vi "CLSUIP_GetOverlayImageData.vi"(2 "error in (no error)":errorcluster, 3 "Access":T1) -> (0 "error out":errorcluster, 1 "image data":T2)   [LabVIEW 2021, in "MemberVICreation.lvlib"]
uses:
  <resource>/Framework/Providers/LVClassLibrary/NewAccessors/MemberVICreation.lvlib
  <vilib>/picture/picture.llb/imagedata.ctl
  <resource>/Framework/Providers/LVClassLibrary/NewAccessors/CLSUIP_Access.ctl
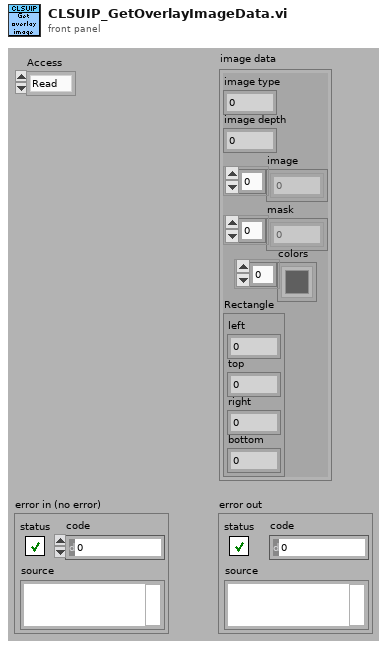
[diagram p1: front panel]
types:
  T1 = typedef "MemberVICreation.lvlib/CLSUIP_Access.ctl" = enum16{"Read", "Write", "R/W"}
  T2 = typedef "imagedata.ctl" = cluster{"image type":i32, "image depth":i32, "image":u8[], "mask":u8[], "colors":u32[], "Rectangle":cluster{"left":i16, "top":i16, "right":i16, "bottom":i16}}
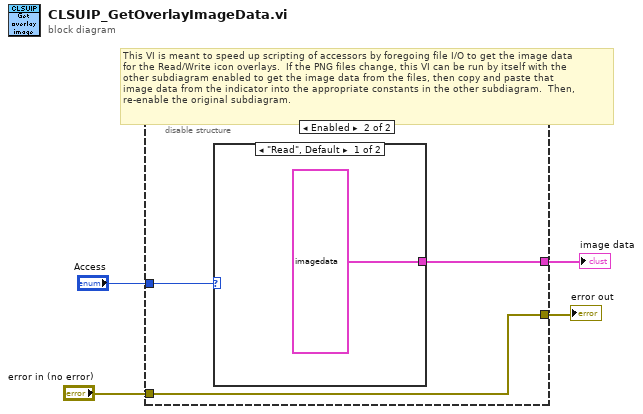
[diagram p0: block diagram]
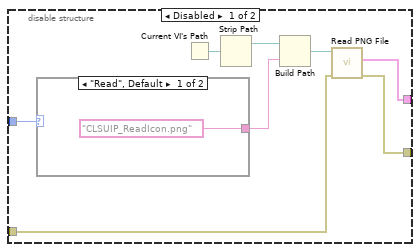
[diagram p2: hidden frame]
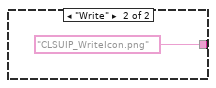
[diagram p3: hidden frame]
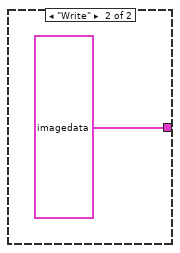
[diagram p4: hidden frame]
diagram:
  # "This VI is meant to speed up scripting of accessors by foregoing file I/O to get the image data\nfor the Read/Write icon overlays.  If the PNG files change, this VI can be run by itself with the\nother subdiagram enabled to get the image data from the files, then copy and paste that\nimage data from the indicator into the appropriate constants in the other subdiagram.  Then,\nre-enable the original subdiagram."
  n1 = disable-structure shown="Enabled" {
    disable-tunnel: [w12 w15] -> w4
    disable-tunnel: [w11 w16] -> w3
    disable-tunnel: "error in (no error)" -> [w9 w15]
    disable-tunnel: "Access" -> [w7 w17]
    frame Disabled {
      n2 = case shown="\"Read\", Default" w7 {
        tunnel: ["CLSUIP_ReadIcon.png" "CLSUIP_WriteIcon.png"] -> w8
        frame "Read", Default {
        }
        frame "Write" {
        }
      }
      n3 = Current VI's Path() -> (path=w5:path)
      n4 = Strip Path(path=w5) -> (stripped path=w6:path)  [unwired: 1 out]
      n5 = Build Path(base path=w6, name or relative path=w8) -> (appended path=w10:path)
      n6 = call <vilib>:"Read PNG File.vi"("error in (no error)"=w9, "path to PNG file"=w10) -> ("error out"=w12:errorcluster, "image data"=w11:T2)  [unwired: 7 in, 1 out]
    }
    frame Enabled {
      n7 = case shown="\"Read\", Default" w17 {
        tunnel: [T2 {"image type"=0, "image depth"=24, "image"=[255, 255, 255, 255, 255, 255, 255, 255, 255, 255, 255, 255, 255, 255, 255, 0, 0, 0, 0, 0, 0, 255, 255, 255, 255, 255, 255, 255, 255, 255, 255, 255, 255, 255, 255, 255, 255, 255, 255, 0, 0, 0, 0, 0, 0, 255, 255, 255, 255, 255, 255, 255, 255, 255, 255, 255, 255, 255, 255, 255, 0, 0, 0, 255, 255, 255, 255, 255, 255, 0, 0, 0, 255, 255, 255, 255, 255, 255, 255, 255, 255, 255, 255, 255, 0, 0, 0, 255, 255, 255, 255, 255, 255, 0, 0, 0, 255, 255, 255, 255, 255, 255, 255, 255, 255, 0, 0, 0, 255, 255, 255, 255, 255, 255, 255, 255, 255, 0, 0, 0, 255, 255, 255, 255, 255, 255, 255, 255, 255, 0, 0, 0, 255, 255, 255, 255, 255, 255, 255, 255, 255, 0, 0, 0, 255, 255, 255, 255, 255, 255, 0, 0, 0, 0, 0, 0, 255, 255, 255, 255, 255, 255, 255, 255, 255, 255, 255, 255, 255, 255, 255, 255, 255, 255, 0, 0, 0, 0, 0, 0, 255, 255, 255, 255, 255, 255, 255, 255, 255, 255, 255, 255, 255, 255, 255, 0, 0, 0, 255, 255, 255, 255, 255, 255, 0, 0, 0, 255, 255, 255, 0, 0, 0, 0, 0, 0, 255, 255, 255, 0, 0, 0, 255, 255, 255, 0, 255, 255, 0, 0, 0, 255, 255, 255, 255, 255, 255, 255, 255, 255, 0, 0, 0, 255, 255, 255, 255, 255, 255, 0, 255, 255, 0, 255, 255, 0, 0, 0, 255, 255, 255, 255, 255, 255, 0, 0, 0, 255, 255, 255, 255, 255, 255, 255, 255, 255, 0, 255, 255, 0, 0, 0, 255, 255, 255, 255, 255, 255, 0, 0, 0, 0, 255, 255, 255, 255, 255, 0, 255, 255, 0, 214, 214, 0, 0, 0, 255, 255, 255, 255, 255, 255, 0, 0, 0, 0, 255, 255, 255, 255, 255, 0, 255, 255, 0, 214, 214, 0, 0, 0, 255, 255, 255, 255, 255, 255, 255, 255, 255, 0, 0, 0, 0, 255, 255, 0, 255, 255, 0, 0, 0, 255, 255, 255, 255, 255, 255, 255, 255, 255, 255, 255, 255, 0, 0, 0, 0, 255, 255, 0, 214, 214, 0, 0, 0, 255, 255, 255, 255, 255, 255, 255, 255, 255, 255, 255, 255, 255, 255, 255, 0, 0, 0, 0, 0, 0, 255, 255, 255, 255, 255, 255, 255, 255, 255, 255, 255, 255, 255, 255, 255, 255, 255, 255, 0, 0, 0, 0, 0, 0, 255, 255, 255, 255, 255, 255, 255, 255, 255, 255, 255, 255, 255, 255, 255, 255, 255, 255, 255, 255, 255, 255, 255, 255, 255, 255, 255, 255, 255, 255, 255, 255, 255, 255, 255, 255, 255, 255, 255, 255, 255, 255, 255, 255, 255, 255, 255, 255, 255, 255, 255, 255, 255, 255, 255, 255, 255, 255, 255, 255, 255, 255, 255, 255, 255, 255, 255, 255, 255, 255, 255, 255, 255, 255, 255, 255, 255, 255, 255, 255, 255, 255, 255, 255, 255, 255, 255, 255, 255, 255, 255, 255, 255, 255, 255, 255, 255, 255, 255, 255, 255, 255, 255, 255, 255, 255, 255, 255, 255, 255, 255, 255, 255, 255, 255, 255, 255, 255, 255, 255, 255, 255, 255, 255, 255, 255, 255, 255, 255, 255, 255, 255, 255, 255, 255, 255, 255, 255, 255, 255, 255, 255, 255, 255, 255, 255, 255, 255, 255, 255, 255, 255, 255, 255, 255, 255, 255, 255, 255, 255, 255, 255, 255, 255, 255, 255, 255, 255, 255, 255, 255, 255, 255, 255, 255, 255, 255, 255, 255, 255, 255, 255, 255, 255, 255, 255, 255, 255, 255, 255, 255, 255, 255, 255, 255, 255, 255, 255, 255, 255, 255, 255, 255, 255], "mask"=[], "colors"=[], "Rectangle"={"left"=0, "top"=0, "right"=16, "bottom"=13}} ("image subset") T2 {"image type"=0, "image depth"=8, "image"=[0, 0, 0, 0, 1, 1, 1, 1, 0, 0, 0, 0, 0, 0, 1, 3, 3, 3, 1, 0, 0, 0, 0, 1, 3, 3, 3, 3, 1, 0, 0, 0, 0, 1, 1, 3, 3, 1, 0, 0, 0, 0, 1, 2, 2, 1, 1, 1, 0, 0, 0, 0, 1, 2, 2, 2, 1, 0, 0, 0, 0, 1, 2, 2, 2, 2, 1, 0, 0, 0, 0, 1, 2, 2, 2, 1, 0, 0, 0, 0, 1, 2, 2, 2, 2, 1, 0, 0, 0, 0, 1, 2, 2, 2, 1, 0, 0, 0, 0, 0, 1, 1, 2, 2, 1, 0, 0, 0, 0, 0, 1, 1, 1, 1, 0, 0, 0, 0, 0, 0, 1, 1, 1, 0, 0, 0, 0, 0, 0, 0, 1, 1, 0, 0, 0, 0, 0, 0, 0, 0, 1, 0, 0, 0, 0, 0, 0, 0, 0, 0], "mask"=[], "colors"=[16777215, 0, 16776960, 16711935, 0, 0, 0, 0, 0, 0, 0, 0, 0, 0, 0, 0, 0, 0, 0, 0, 0, 0, 0, 0, 0, 0, 0, 0, 0, 0, 0, 0, 0, 0, 0, 0, 0, 0, 0, 0, 0, 0, 0, 0, 0, 0, 0, 0, 0, 0, 0, 0, 0, 0, 0, 0, 0, 0, 0, 0, 0, 0, 0, 0, 0, 0, 0, 0, 0, 0, 0, 0, 0, 0, 0, 0, 0, 0, 0, 0, 0, 0, 0, 0, 0, 0, 0, 0, 0, 0, 0, 0, 0, 0, 0, 0, 0, 0, 0, 0, 0, 0, 0, 0, 0, 0, 0, 0, 0, 0, 0, 0, 0, 0, 0, 0, 0, 0, 0, 0, 0, 0, 0, 0, 0, 0, 0, 0, 0, 0, 0, 0, 0, 0, 0, 0, 0, 0, 0, 0, 0, 0, 0, 0, 0, 0, 0, 0, 0, 0, 0, 0, 0, 0, 0, 0, 0, 0, 0, 0, 0, 0, 0, 0, 0, 0, 0, 0, 0, 0, 0, 0, 0, 0, 0, 0, 0, 0, 0, 0, 0, 0, 0, 0, 0, 0, 0, 0, 0, 0, 0, 0, 0, 0, 0, 0, 0, 0, 0, 0, 0, 0, 0, 0, 0, 0, 0, 0, 0, 0, 0, 0, 0, 0, 0, 0, 0, 0, 0, 0, 0, 0, 0, 0, 0, 0, 0, 0, 0, 0, 0, 0, 0, 0, 0, 0, 0, 0, 0, 0, 0, 0, 0, 0, 0, 0, 0, 0, 0, 0, 0, 0, 0, 0, 0, 0], "Rectangle"={"left"=0, "top"=0, "right"=9, "bottom"=15}} ("image data")] -> w16
        frame "Read", Default {
        }
        frame "Write" {
        }
      }
    }
  }
  "error out" <- w4
  "image data" <- w3
